vi "Test Variant.vi"() -> ()   [LabVIEW 2020, in "Linearisierung v2.lvlib" / "Gasteiler.lvlib" / "HovaCAL_Interface.lvlib"]
uses:
  HovaCAL_Interface.lvlib
panel:
  in  "MFC Gasauswahl 2":u16[](array[ring]) caption="MFC Gasauswahl" items=["AIR"]
  in  "MFC3 Gasauswahl Array":u16(ring) caption="MFC Gasauswahl" items=["AIR", "N2"]
  in  "MFC2 Gasauswahl Array":u16(ring) caption="MFC Gasauswahl" items=["AIR", "O2"]
  in  "Map":map{string, i32}(c390)
  in  "Set":set{string}(c389)
  out "Variant 2":variant
  in  "LabVIEW-Objekt":refnum<class>
  in  "MFC1 Gasauswahl Array":u16(ring) caption="MFC Gasauswahl" items=["AIR"]
  in  "MFC Gasauswahl":u16[](array[ring]) items=["AIR"]
  out "Variant":variant
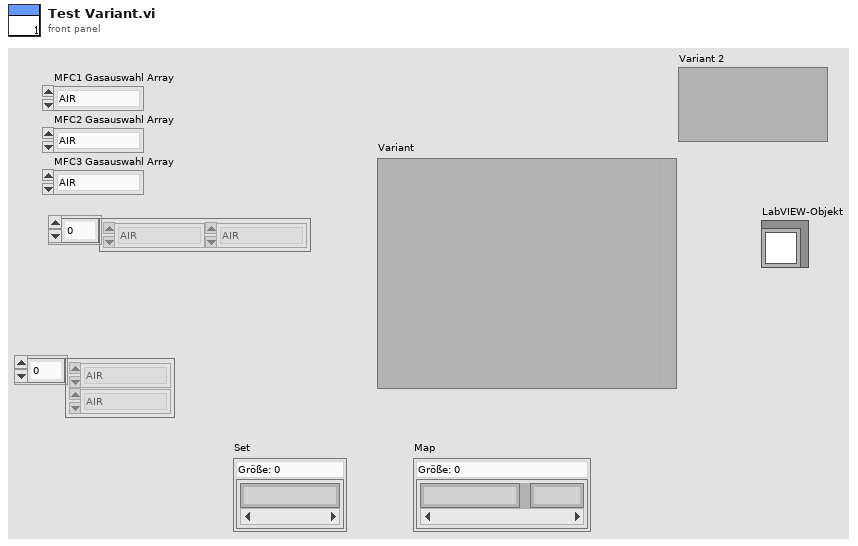
[diagram p1: front panel]
types:
  T1 = typedef "LVStringsAndValuesArrayTypeDef_U16.ctl" = cluster{"String":string, "Value":u16}[]
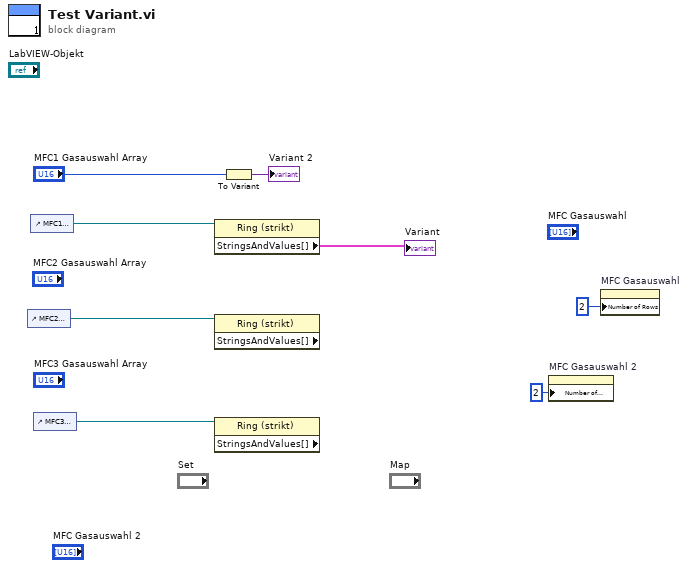
[diagram p0: block diagram]
diagram:
  n1 = control-ref of="MFC2 Gasauswahl Array"() -> (w5:refnum<vi>)
  n2 = control-ref of="MFC1 Gasauswahl Array"() -> (w6:refnum<vi>)
  n3 = control-ref of="MFC3 Gasauswahl Array"() -> (w4:refnum<vi>)
  n4 = property class="Ring (strikt)"(reference=w6) -> ("StringsAndValues[]"=→"Variant":T1)  [unwired: 1 in, 2 out]
  n5 = property class="Ring (strikt)" props=["StringsAndValues[]"](reference=w5) -> ()  [unwired: 1 in, 3 out]
  n6 = property class="Ring (strikt)" props=["StringsAndValues[]"](reference=w4) -> ()  [unwired: 1 in, 3 out]
  n7 = To Variant(anything="MFC1 Gasauswahl Array") -> (Variant=→"Variant 2":variant)
  n8 = property on="MFC Gasauswahl 2" class="Arr (strikt)"("Number of Columns"=u32 2 ("Zeilenanzahl")) -> ()  [unwired: 2 in, 2 out]
  n9 = property on="MFC Gasauswahl" class="Arr (strikt)"("Number of Rows"=u32 2 ("Spaltenanzahl")) -> ()  [unwired: 2 in, 2 out]
